vi "ISO String To Timestamp.vi"(8 "error in (no error)":errorcluster, 11 "ISO Timestamp String":string) -> (0 "error out":errorcluster, 3 "Time Stamp":timestamp)   [LabVIEW 2019, in "JKI JSON Serialization.lvlib" / "JSON Deserializer.lvclass"]
doc: "Converts ISO formatted timestamp string to a LabVIEW timestamp.\n\nJKI JSON 1.1.10.37\nTomi Maila - JKI\nCopyright (c) 2017, JKI"
uses:
  JSON Deserializer.lvclass
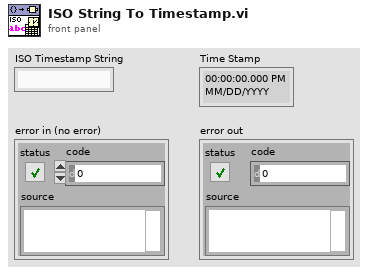
[diagram p1: front panel]
types:
  T1 = typedef "LVDateTimeRec.ctl" = cluster{"fractional second":dbl, "second":i32, "minute":i32, "hour":i32, "day of month":i32, "month":i32, "year":i32, "day of week":i32, "day of year":i32, "DST":i32}
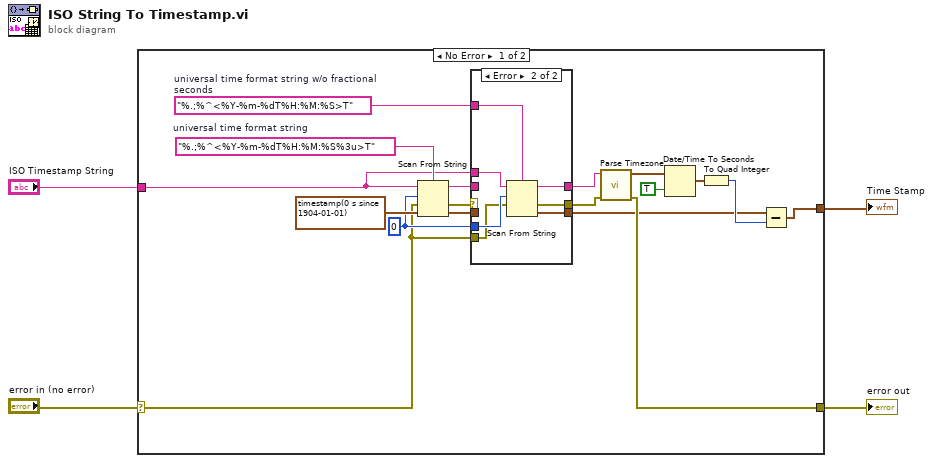
[diagram p0: block diagram]
diagram:
  n1 = case shown="No Error" "error in (no error)" {
    selector: "error in (no error)" -> [w5 w33]
    tunnel: [w22 _] -> w4
    tunnel: [w17 w33] -> w3
    tunnel: "ISO Timestamp String" -> [w9 _]
    frame No Error {
      w7 = "%.;%^<%Y-%m-%dT%H:%M:%S>T"  # universal time format string w/o fractional seconds
      w8 = u32 0 ("initial scan location")
      w15 = "%.;%^<%Y-%m-%dT%H:%M:%S%3u>T"  # universal time format string
      n2 = Scan From String(format string=w15, input string=w9, initial scan location=w8, error in=w5, default 1=timestamp(0 s since 1904-01-01) ("default value 1")) -> (remaining string=w13:string, error out=w14:errorcluster, output 1=w11:timestamp)  [unwired: 1 out]
      n3 = case shown="Error" w14 {
        selector: w14 -> [w24 _]
        tunnel: w13 -> [w25 _]
        tunnel: [w25 w28] -> w12
        tunnel: w11 -> [w23 _]
        tunnel: [w24 w27] -> w10
        tunnel: w5 -> [_ w30]
        tunnel: w9 -> [_ w32]
        tunnel: w8 -> [_ w31]
        tunnel: w7 -> [_ w29]
        tunnel: [w23 w26] -> w6
        frame No Error {
        }
        frame Error {
          n4 = Scan From String(format string=w29, input string=w32, initial scan location=w31, error in=w30) -> (remaining string=w28:string, error out=w27:errorcluster, output 1=w26:timestamp)  [unwired: 1 in, 1 out]
        }
      }
      n5 = call "Parse Timezone.vi"("error in (no error)"=w10, "Timezone String"=w12) -> ("error out"=w17:errorcluster, "time zone offset"=w18:T1)  [unwired: 8 in]
      n6 = Date/Time To Seconds(1:TRUE ("is UTC (F)"), 2:w18) -> (0:w20:timestamp)
      n7 = To Quad Integer(1:w20) -> (0:w21:i64)
      n8 = Subtract(x=w6, y=w21) -> (x-y=w22:timestamp)
    }
    frame Error {
    }
  }
  "Time Stamp" <- w4
  "error out" <- w3
